vi "Read Drive Operation.vi"(8 "Command Info":T5) -> (0 "Command Info":T5, 1 "SubSystem Data":T1, 2 "Command Timing":cluster{"Start Time (ms)":u32, "Iterations":i32})   [LabVIEW 2019]
doc: "Returns the details about the currently executing command."
uses:
  <vilib>/Rock Robotics/WPI/Framework/Command Status Info.ctl
  <vilib>/Rock Robotics/WPI/Framework/Completion Status.ctl
  <vilib>/Rock Robotics/WPI/Framework/Completion Notifier.ctl
  Implementation/Drive Setpoints.ctl
  Implementation/Drive Operations.ctl
  Bordeaux/Command Stuff/Single Cmd Info.ctl
  <vilib>/picture/picture.llb/imagedata.ctl
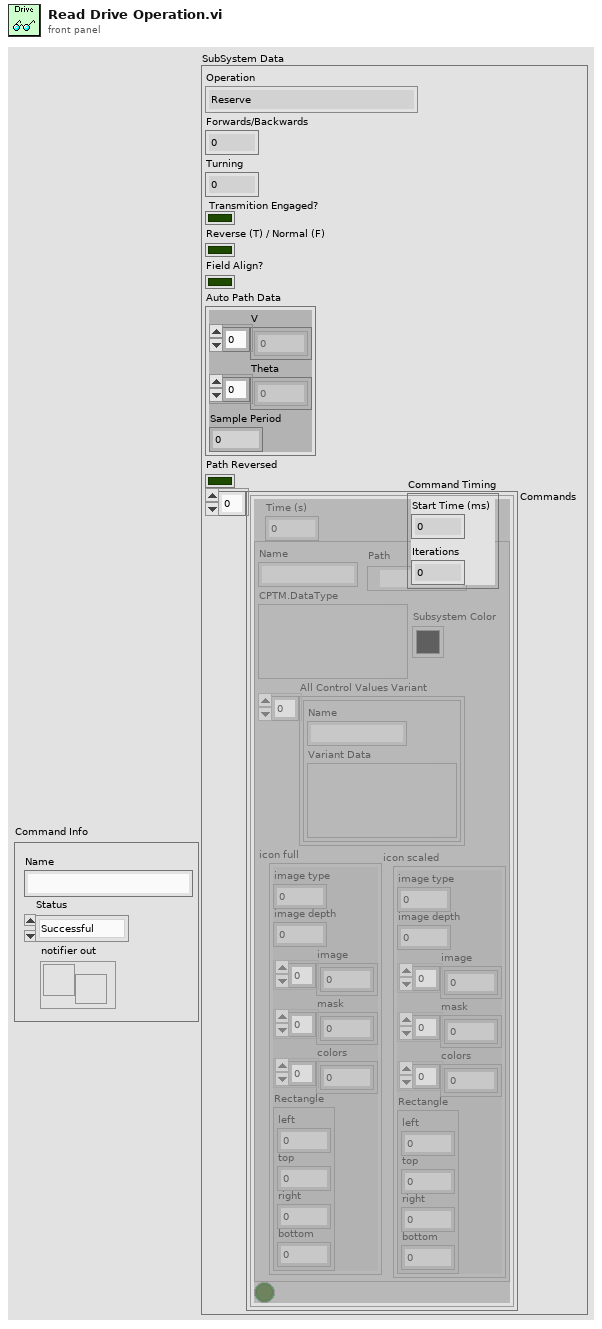
[diagram p1: front panel]
types:
  T1 = typedef "Drive Setpoints.ctl" = cluster{"Operation":T2, "Forwards/Backwards":dbl, "Turning":dbl, "Transmition Engaged?":bool, "Reverse (T) / Normal (F)":bool, "Field Align?":bool, "Auto Path Data":cluster{"V":dbl[], "Theta":dbl[], "Sample Period":dbl}, "Path Reversed":bool, "Commands":cluster{"Time (s)":dbl, T3, bool}[]}
  T2 = typedef "Drive Operations.ctl" = enum16{"Reserve", "Read Current", "Immediate", "Pod Racer", "Ball AA", "Feeder Station AA", "Play Back From Log"}
  T3 = typedef "Single Cmd Info.ctl" = cluster{"Name":string, "CPTM.DataType":variant, "All Control Values Variant":cluster{"Name":string, "Variant Data":variant}[], "icon full":T4, "icon scaled":T4, "Path":path, "Subsystem Color":u32}
  T4 = typedef "imagedata.ctl" = cluster{"image type":i32, "image depth":i32, "image":u8[], "mask":u8[], "colors":u32[], "Rectangle":cluster{"left":i16, "top":i16, "right":i16, "bottom":i16}}
  T5 = typedef "Command Status Info.ctl" = cluster{"Name":string, "Status":T6, "notifier out":T7}
  T6 = typedef "Completion Status.ctl" = enum16{"Successful", "Aborted", "Incomplete"}
  T7 = typedef "Completion Notifier.ctl" = refnum<notifier>
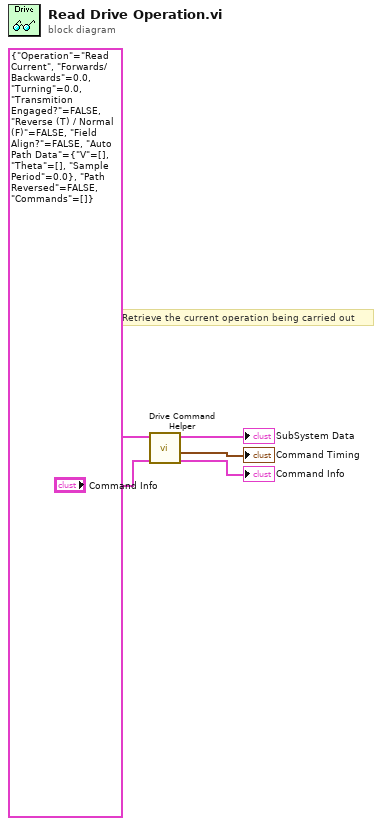
[diagram p0: block diagram]
diagram:
  # "Retrieve the current operation being carried out"
  n1 = call "Drive Command Helper.vi"("Command Info In"="Command Info", "SubSystem Data"=T1 {"Operation"=enum."Read Current", "Forwards/Backwards"=0.0, "Turning"=0.0, "Transmition Engaged?"=FALSE, "Reverse (T) / Normal (F)"=FALSE, "Field Align?"=FALSE, "Auto Path Data"={"V"=[], "Theta"=[], "Sample Period"=0.0}, "Path Reversed"=FALSE, "Commands"=[]}) -> ("Command Info Out"=→"Command Info":T5, "Command Timing"=→"Command Timing":cluster{"Start Time (ms)":u32, "Iterations":i32}, "SubSystem Data"=→"SubSystem Data":T1)  [unwired: 7 in]
